vi "LEP_RV_LaunchDownload.vi"(8 "error in (no error)":errorcluster) -> (0 "error out":errorcluster)   [LabVIEW 2011]
doc: "Runs the embedded application on a console located in the <B>Build Path</B> directory ."
uses:
  <vilib>/LabVIEW Targets/Embedded/ASWServer/MPU_ASWServer_GeneralIcons.ctl
  <vilib>/LabVIEW Targets/Embedded/ASWServer/MPU_ASWServer_GeneralCtrls.ctl
  LEP_RV_LaunchGlobals.vi
  <vilib>/LabVIEW Targets/Embedded/ASWServer/MPU_ASWServer_General_SetProgressBarTitle.vi
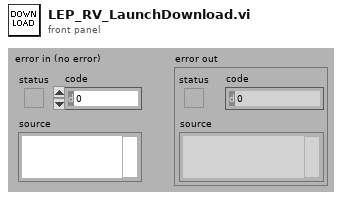
[diagram p1: front panel]
types:
  T1 = typedef "MPU_ASWServer_GeneralIcons.ctl" = enum16{"Complete", "Disconnected", "Error", "Initializing", "Ready", "Running", "Stopped", "Unknown", "No Change"}
  T2 = typedef "MPU_ASWServer_GeneralCtrls.ctl" = enum16{"Build Status", "Download Status", "Target Name", "Target Type", "Application Name"}
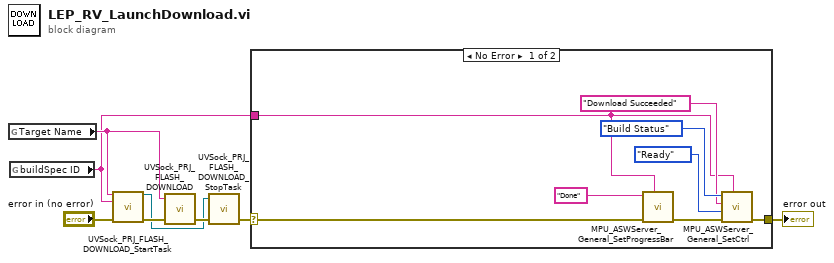
[diagram p0: block diagram]
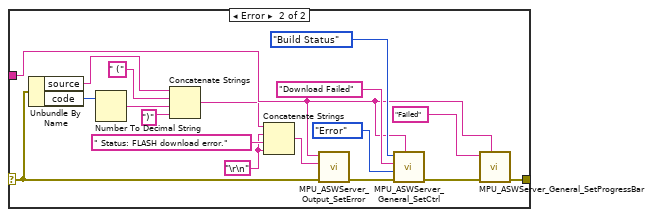
[diagram p2: hidden frame]
diagram:
  n1 = global read "LEP_RV_LaunchGlobals.vi" "Target Name"() -> (w3:string)
  n2 = global read "LEP_RV_LaunchGlobals.vi" "buildSpec ID"() -> (w2:string)
  n3 = call "UVSock_PRJ_FLASH_DOWNLOAD_StartTask.vi"("Target"=w3, "buildSpec ID"=w2, "error in (no error)"="error in (no error)") -> ("Task Done"=w5:refnum<notifier>, "error out"=w7:errorcluster)  [unwired: 11 out]
  n4 = call "UVSock_PRJ_FLASH_DOWNLOAD.vi"("error in (no error)"=w7, "Target"=w3) -> ("error out"=w6:errorcluster)  [unwired: 3 out]
  n5 = call "UVSock_PRJ_FLASH_DOWNLOAD_StopTask.vi"("error in (no error)"=w6, "Task Done"=w5) -> ("error out"=w8:errorcluster)  [unwired: 3 out]
  n6 = case shown="No Error" w8 {
    selector: w8 -> [w12 w28]
    tunnel: [w13 w22] -> w4
    tunnel: w2 -> [w10 w21]
    frame No Error {
      n7 = call-poly <vilib>:"MPU_ASWServer_General_SetProgressBar.vi"("buildSpec ID"=w10, "error in"=w12, "title"="Done") -> ("error out"=w9:errorcluster)  [unwired: 6 in, 2 out]
      n8 = call <vilib>:"MPU_ASWServer_General_SetCtrl.vi"("buildSpec ID"=w10, "error in"=w9, "icon"=MPU_ASWServer_GeneralIcons."Ready", "value"="Download Succeeded", "control"=MPU_ASWServer_GeneralCtrls."Build Status") -> ("error out"=w13:errorcluster)  [unwired: 4 in, 2 out]
    }
    frame Error {
      w17 = "\r\n"
      n9 = Unbundle By Name(w28) -> ("source"=w31:string, "code"=w30:i32)
      n10 = Number To Decimal String(number=w30) -> (decimal integer string=w34:string)  [unwired: 1 out]
      n11 = Concatenate Strings(w31, " (" ("string"), w34, ")" ("string")) -> (w19:string)
      n12 = Concatenate Strings(w19, w17, " Status: FLASH download error." ("title"), w17) -> (w29:string)
      n13 = call <vilib>:"MPU_ASWServer_Output_SetError.vi"("error in"=w28, "error str"=w29, "buildSpec ID"=w21) -> ("error out"=w27:errorcluster)  [unwired: 6 in]
      n14 = call <vilib>:"MPU_ASWServer_General_SetCtrl.vi"("buildSpec ID"=w21, "error in"=w27, "icon"=MPU_ASWServer_GeneralIcons."Error", "value"="Download Failed", "control"=MPU_ASWServer_GeneralCtrls."Build Status") -> ("error out"=w23:errorcluster)  [unwired: 4 in, 2 out]
      n15 = call-poly <vilib>:"MPU_ASWServer_General_SetProgressBar.vi"("buildSpec ID"=w21, "error in"=w23, "title"="Failed") -> ("error out"=w22:errorcluster)  [unwired: 6 in, 2 out]
    }
  }
  "error out" <- w4
